vi "update.description.request.vi"(8 "error in":errorcluster, 11 "Description":string) -> (0 "error out":errorcluster, 1 "Request":string)   [LabVIEW 2020, in "Run.lvclass"]
uses:
  Run.lvclass
  <vilib>/JDP Science/JSONtext/LVClass Serializer/JSONtext LVClass Serializer.lvclass
  4393078b-8c31-48a1-905f-a31b045981fd.vi
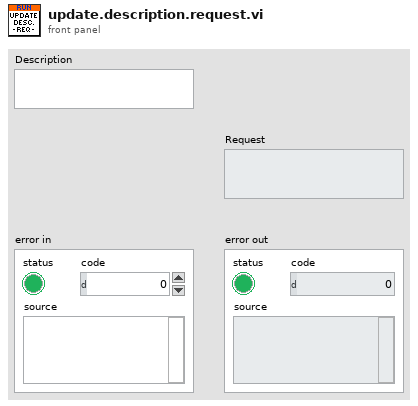
[diagram p1: front panel]
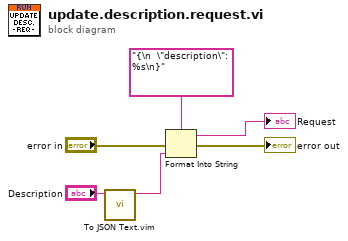
[diagram p0: block diagram]
diagram:
  n1 = call "To JSON Text.vim"("Anything"="Description") -> ("<JSON>"=w1:string)  [unwired: 9 in, 1 out]
  n2 = Format Into String(format string="{\n  \"description\": %s\n}", error in="error in", w1) -> (resulting string=→"Request":string, error out=→"error out":errorcluster)  [unwired: 1 in]
